vi "Config.vi"() -> ()   [LabVIEW 2020]
uses:
  Global_Variable/A131258.vi
  Global_Variable/Global.vi
  Database/Global1.vi
  <vilib>/Utility/config.llb/NI_LVConfig.lvlib
panel:
  in  "工位选择":cluster{"左工位":bool, "右工位":bool}
  in  "系数":bool
  in  "产品型号":string(combo)
  in  "删除":bool
  in  "确定":bool
  in  "添加":bool
  in  "退出":bool
  in  "更新":bool
  in  "选项卡控件":enum32{"产品参数", "系统参数"}(tab)
  in  "判定框范围":string[][](table)=[["°"], ["N"], ["°"], ["N"], ["°"], ["N"], ["°"], ["N"]]
  in  "结果判定参数":string[][](table)=[["N"], ["N"], ["N"], ["N"], ["N"], ["N"], ["N"], ["N"], ["N"]]
  in  "工位滤波":cluster{"启用滤波":bool, "滤波系数":dbl}
  in  "系统参数设置":string[][](table)=[[""], [""], [""], [""]]
  # "上下柱管总成压装"
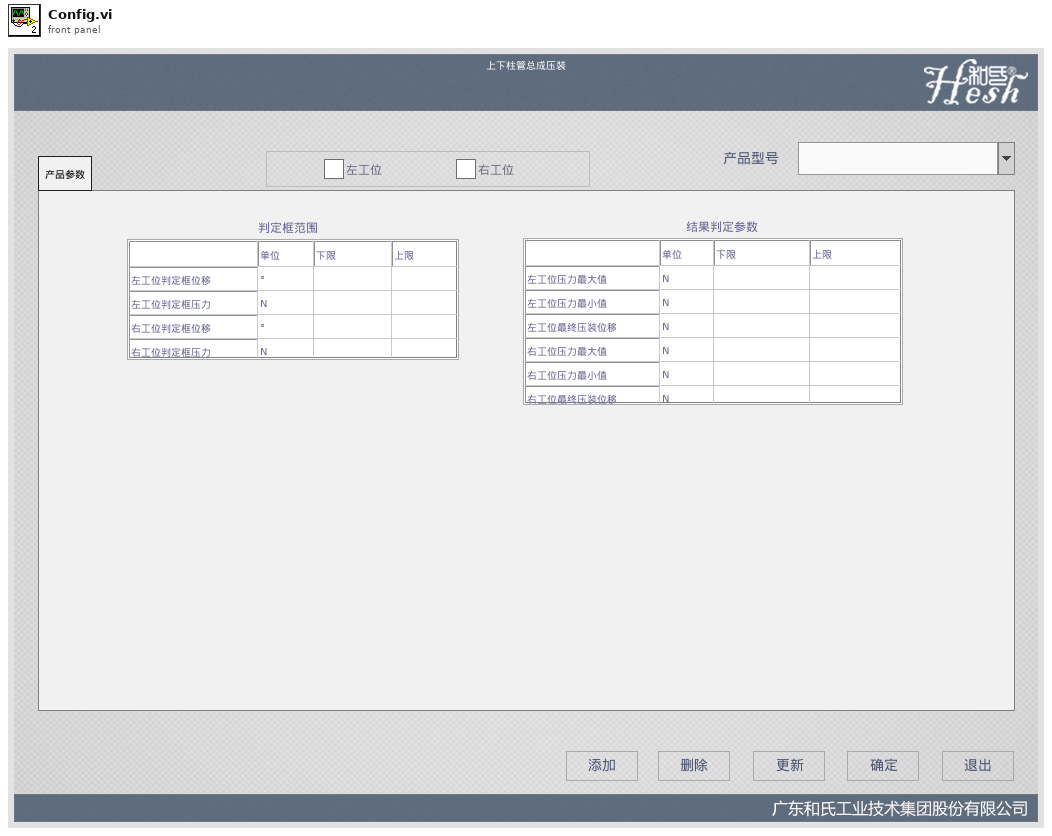
[diagram p1: front panel]
types:
  T1 = typedef "NI_LVConfig.lvlib/Config Data RefNum.ctl" = refnum<k1>
  T2 = cluster{"用户编号":string, "用户名":string, "用户密码(密文)":string, "用户权限":string}
  T3 = cluster{"[0]":cluster{string, dbl, dbl}, "[1]":cluster{string, dbl, dbl}}
  T4 = cluster{"[0]":cluster{string, dbl, dbl}, "[1]":cluster{string, dbl, dbl}, "[2]":cluster{string, dbl, dbl}}
  T5 = cluster{"X ":cluster{"单位":string, "下限":dbl, "上限":dbl}, "Y":cluster{"单位":string, "下限":dbl, "上限":dbl}}
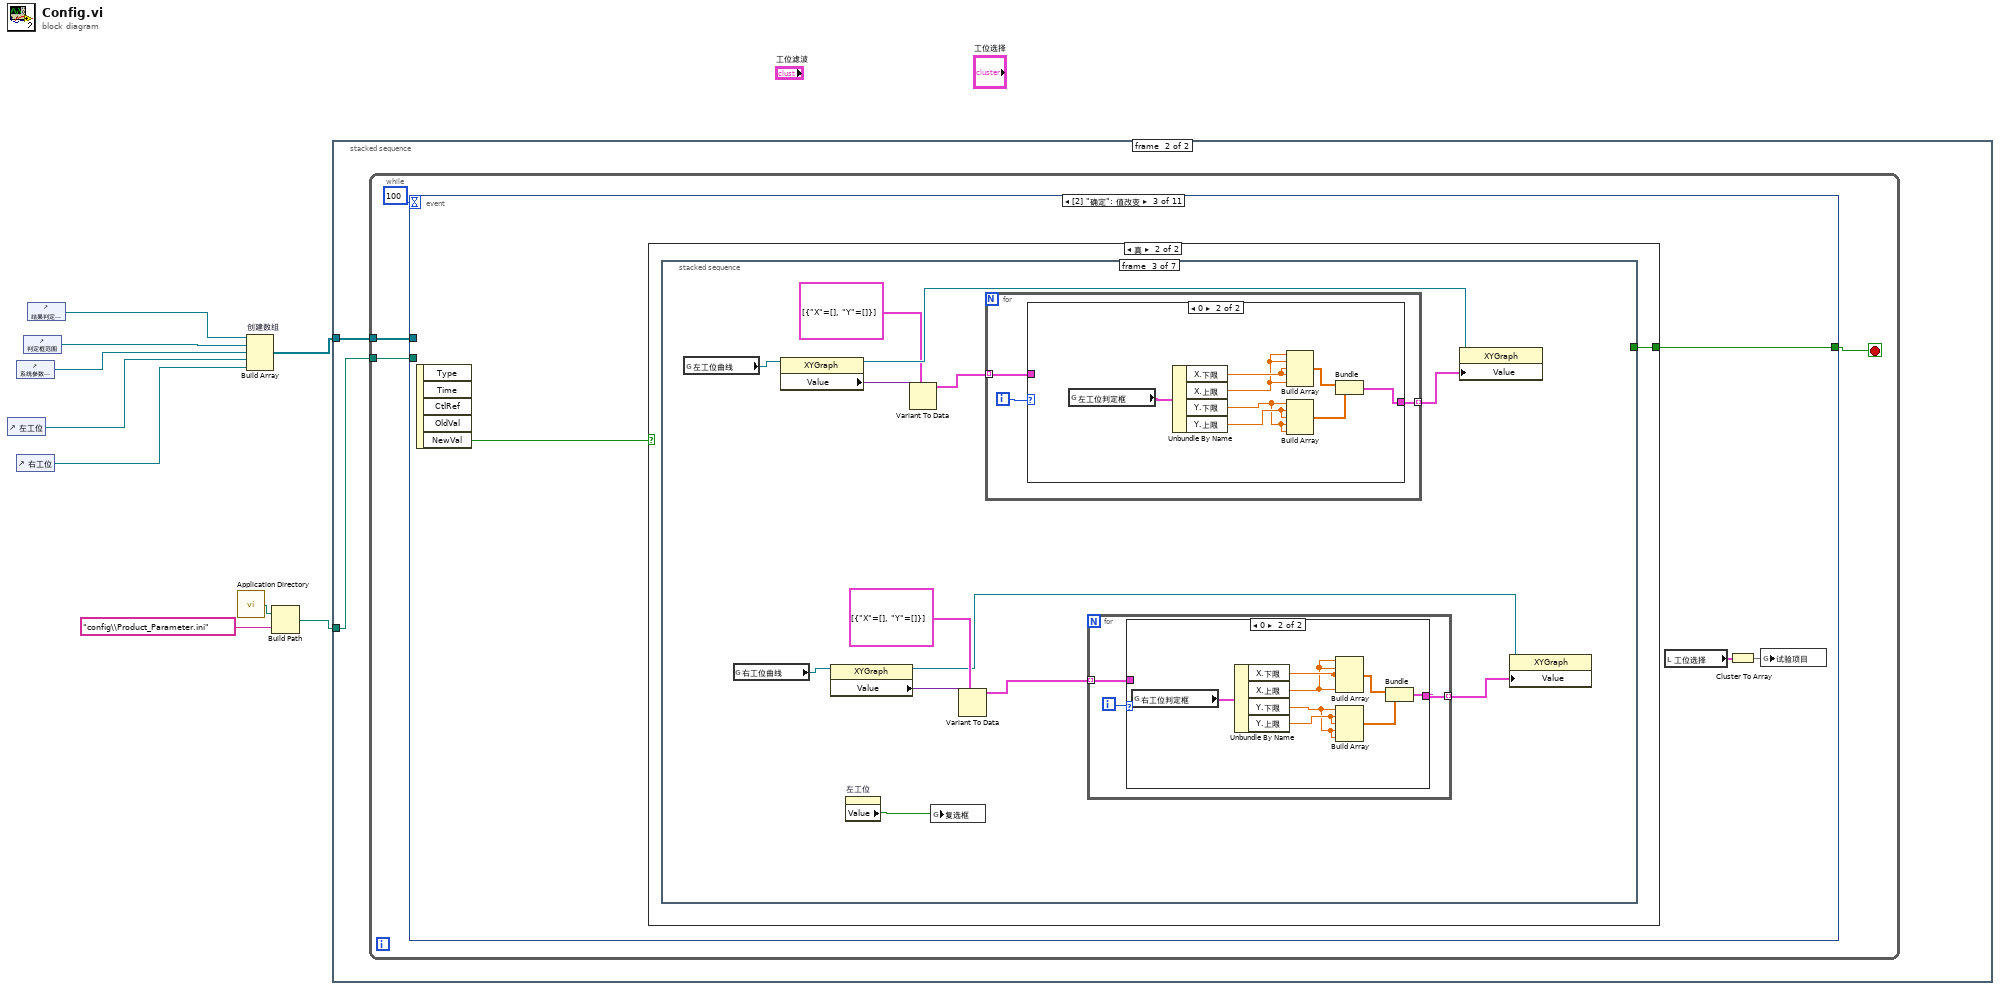
[diagram p0: block diagram]
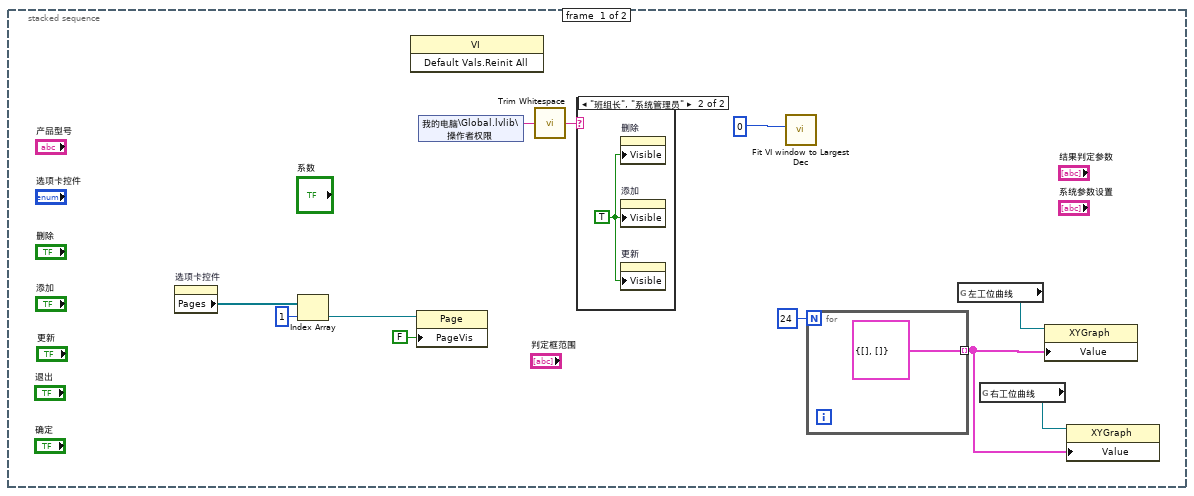
[diagram p2: hidden frame]
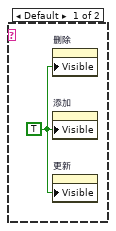
[diagram p3: hidden frame]
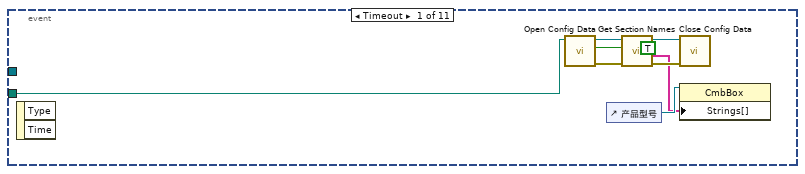
[diagram p4: hidden frame]
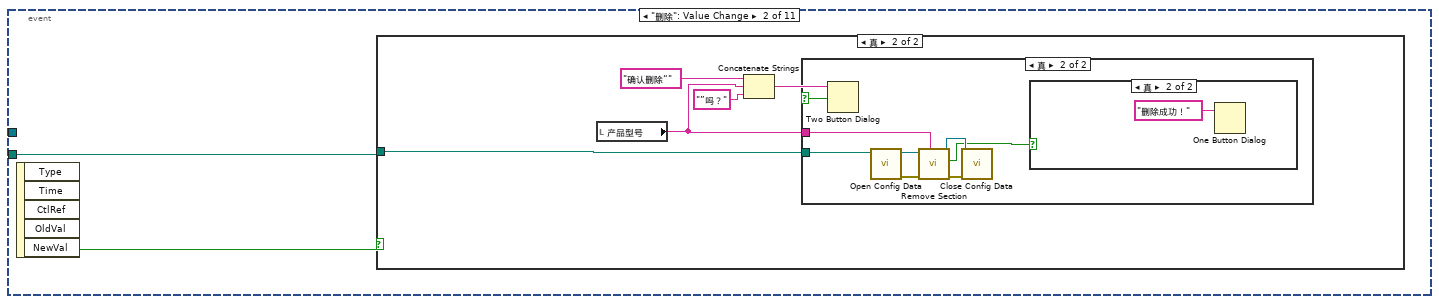
[diagram p5: hidden frame]
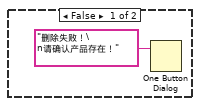
[diagram p8: hidden frame]
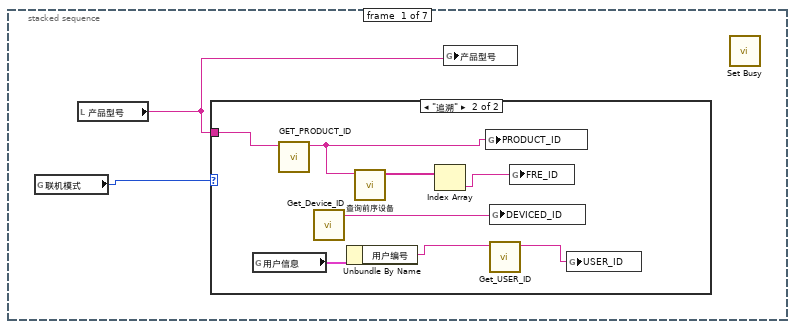
[diagram p10: hidden frame]
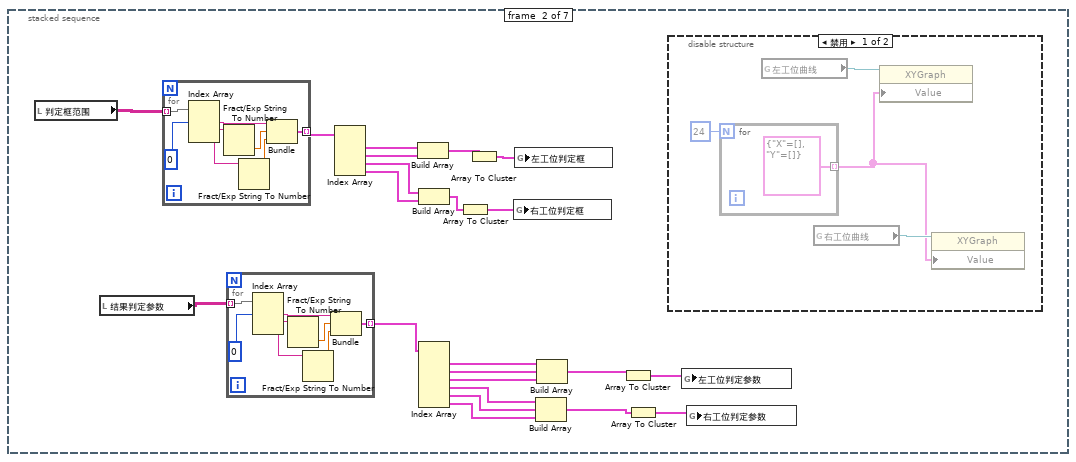
[diagram p12: hidden frame]
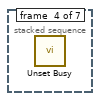
[diagram p16: hidden frame]
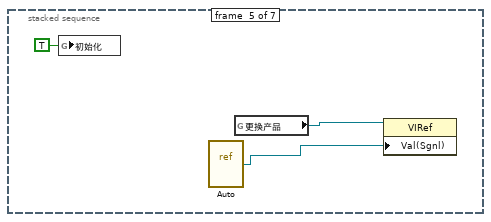
[diagram p17: hidden frame]
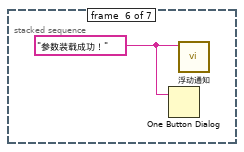
[diagram p18: hidden frame]
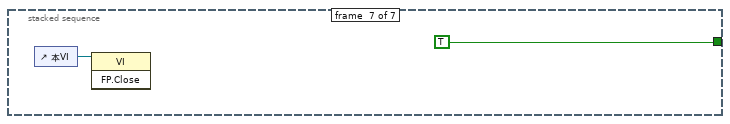
[diagram p19: hidden frame]
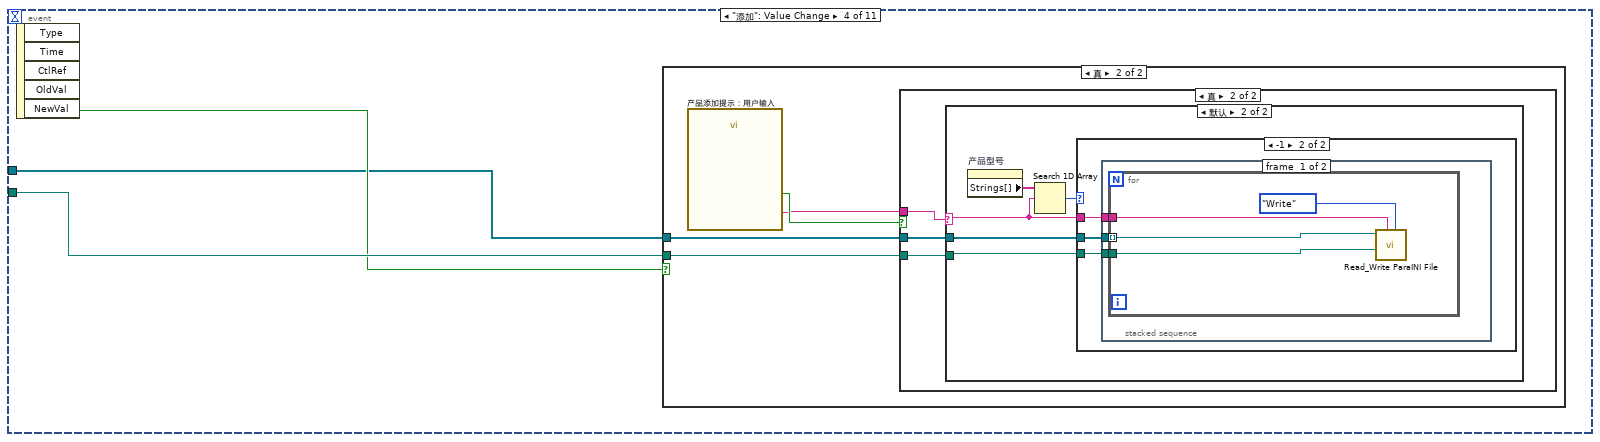
[diagram p20: hidden frame]
diagram:
  n1 = control-ref of="左工位"() -> (w2:refnum<vi>)
  n2 = control-ref of="系统参数设置"() -> (w6:refnum<vi>)
  n3 = control-ref of="右工位"() -> (w1:refnum<vi>)
  n4 = control-ref of="判定框范围"() -> (w3:refnum<vi>)
  n5 = control-ref of="结果判定参数"() -> (w5:refnum<vi>)
  n6 = call <vilib>:"Application Directory.vi"() -> ("Application Directory"=w8:path)
  n7 = Build Array "创建数组"(w5, w3, w6, w2, w1) -> (w9:refnum<vi>[])
  n8 = Build Path(base path=w8, name or relative path="config\\Product_Parameter.ini" ("名称或相对路径")) -> (appended path=w7:path)
  n9 = stacked-sequence {
    tunnel: w9 -> [_ w24]
    tunnel: w7 -> [_ w25]
    frame #0 {
      n10 = property on="选项卡控件" class="TabCtl (严格)"() -> ("Pages"=w16:refnum<vi>[])  [unwired: 2 in, 2 out]
      n11 = Index Array(array=w16, index=1 ("索引")) -> (element=w17:refnum<vi>)
      n12 = invoke class="VI" method="Default Vals.Reinit All"() -> ()  [unwired: 3 in, 3 out]
      n13 = property class="Page"(reference=w17, "PageVis"=FALSE ("选项卡可见")) -> ()  [unwired: 1 in, 2 out]
      n14 = shared-variable "我的电脑\\Global.lvlib\\操作者权限"() -> (w20:string)  [unwired: 1 in, 1 out]
      n15 = call <vilib>:"Trim Whitespace.vi"("string"=w20) -> ("trimmed string"=w19:string)  [unwired: 1 in]
      n16 = case shown="\"班组长\", \"系统管理员\"" w19 {
        frame Default {
          w22 = TRUE ("可见")
          n17 = property on="删除" class="Bool (严格)"("Visible"=w22) -> ()  [unwired: 2 in, 2 out]
          n18 = property on="添加" class="Bool (严格)"("Visible"=w22) -> ()  [unwired: 2 in, 2 out]
          n19 = property on="更新" class="Bool (严格)"("Visible"=w22) -> ()  [unwired: 2 in, 2 out]
        }
        frame "班组长", "系统管理员" {
          w23 = TRUE ("可见")
          n20 = property on="删除" class="Bool (严格)"("Visible"=w23) -> ()  [unwired: 2 in, 2 out]
          n21 = property on="添加" class="Bool (严格)"("Visible"=w23) -> ()  [unwired: 2 in, 2 out]
          n22 = property on="更新" class="Bool (严格)"("Visible"=w23) -> ()  [unwired: 2 in, 2 out]
        }
      }
      n23 = call "Fit VI window to Largest Dec.vi"("border spacing (2 px)"=0) -> ()  [unwired: 5 in, 2 out]
      n24 = for {
        N: 24 -> [_]
        tunnel: [cluster{dbl[], dbl[]} {[], []}] -> w10 mode=indexing
      }
      n25 = global read "A131258.vi" "左工位曲线"() -> (w12:refnum<vi>)
      n26 = global read "A131258.vi" "右工位曲线"() -> (w11:refnum<vi>)
      n27 = property class="XYGraph"(reference=w12, "Value"=w10) -> ()  [unwired: 1 in, 2 out]
      n28 = property class="XYGraph"(reference=w11, "Value"=w10) -> ()  [unwired: 1 in, 2 out]
    }
    frame #1 {
      n29 = while {
        tunnel: w25 -> [w29]
        tunnel: w24 -> [w26]
        stop <- w28 stop-if-true
        n30 = event shown="[2] \"确定\": 值改变" {
          selector: _ -> [_ _ _ _ _ _ _ _ _ _ _]
          dyn-events: _ -> [_ _ _ _ _ _ _ _ _ _ _]
          timeout: 100 -> [_ _ _ _ _ _ _ _ _ _ _]
          tunnel: w29 -> [w30 w39 _ w158 w186 _ w209 _ _ _ _]
          tunnel: [_ _ w57 _ _ TRUE _ _ _ _ TRUE] -> w28
          tunnel: w26 -> [_ _ _ w156 w184 _ w207 _ _ _ _]
          event Timeout {
            n31 = event-data() -> ()  [unwired: 1 in, 2 out]
            n32 = call <vilib>:"Open Config Data.vi"("create file if necessary (T)"=TRUE, "configuration file path"=w30) -> ("error out"=w34:errorcluster, "refnum"=w33:T1)  [unwired: 7 in, 1 out]
            n33 = control-ref of="产品型号"() -> (w32:refnum<vi>)
            n34 = call <vilib>:"Get Section Names.vi"("error in (no error)"=w34, "refnum"=w33) -> ("error out"=w36:errorcluster, "section names"=w31:string[], "refnum out"=w35:T1)  [unwired: 7 in]
            n35 = call <vilib>:"Close Config Data.vi"("error in (no error)"=w36, "refnum"=w35) -> ()  [unwired: 8 in, 2 out]
            n36 = property on="属性节点" class="CmbBox"(reference=w32, "Strings[]"=w31) -> ()  [unwired: 1 in, 2 out]
          }
          event "删除": Value Change {
            n37 = event-data() -> ("NewVal"=w38:bool)  [unwired: 1 in, 4 out]
            n38 = case shown="真" w38 {
              tunnel: w39 -> [_ w41]
              frame False {
              }
              frame True {
                n39 = local read "产品型号"() -> (w40:string)
                n40 = Concatenate Strings("确认删除“", w40, "”吗？") -> (w43:string)
                n41 = Two Button Dialog(message=w43) -> (T button?=w42:bool)  [unwired: 2 in]
                n42 = case shown="真" w42 {
                  tunnel: w41 -> [_ w47]
                  tunnel: w40 -> [_ w46]
                  frame False {
                  }
                  frame True {
                    n43 = call <vilib>:"Open Config Data.vi"("configuration file path"=w47) -> ("error out"=w49:errorcluster, "refnum"=w52:T1)  [unwired: 8 in, 1 out]
                    n44 = call <vilib>:"Remove Section.vi"("section"=w46, "error in (no error)"=w49, "refnum"=w52) -> ("error out"=w51:errorcluster, "section exists?"=w48:bool, "refnum out"=w50:T1)  [unwired: 6 in]
                    n45 = call <vilib>:"Close Config Data.vi"("error in (no error)"=w51, "refnum"=w50) -> ()  [unwired: 8 in, 2 out]
                    n46 = case shown="真" w48 {
                      frame False {
                        n47 = One Button Dialog(message="删除失败！\n请确认产品存在！" ("消息")) -> ()  [unwired: 1 in, 1 out]
                      }
                      frame True {
                        n48 = One Button Dialog(message="删除成功！" ("消息")) -> ()  [unwired: 1 in, 1 out]
                      }
                    }
                  }
                }
              }
            }
          }
          event "确定": Value Change {
            n49 = event-data() -> ("NewVal"=w58:bool)  [unwired: 1 in, 4 out]
            n50 = case shown="真" w58 {
              tunnel: [_ w59] -> w57
              frame False {
              }
              frame True {
                n51 = stacked-sequence {
                  tunnel: [_ _ _ _ _ _ TRUE] -> w59
                  frame #0 {
                    n52 = global read "Global1.vi" "联机模式"() -> (w61:enum16{"单机", "追溯"})
                    n53 = local read "产品型号"() -> (w60:string)
                    n54 = case shown="\"追溯\"" w61 {
                      tunnel: w60 -> [_ w69]
                      frame "单机", Default {
                      }
                      frame "追溯" {
                        n55 = global read "Global1.vi" "用户信息"() -> (w67:T2)
                        n56 = call "GET_PRODUCT_ID.vi"("PRODFUCT_NAME"=w69) -> ("PRODUCT_ID"=w65:string)  [unwired: 10 in]
                        n57 = call "Get_Device_ID.vi"() -> ("Device_ID"=w63:string)  [unwired: 10 in, 1 out]
                        n58 = Unbundle By Name(w67) -> ("用户编号"=w66:string)
                        n59 = call "查询前序设备.vi"("PRODUCT_ID"=w65) -> ("前序工位"=w68:string[])  [unwired: 10 in]
                        n60 = Index Array(array=w68) -> (element=w64:string)  [unwired: 1 in]
                        n61 = global write "Global.vi" "PRODUCT_ID"(w65) -> ()
                        n62 = global write "Global.vi" "DEVICED_ID"(w63) -> ()
                        n63 = call "Get_USER_ID.vi"("USER_EMPLOYEE_ID"=w66) -> ("USER_ID"=w62:string)  [unwired: 9 in, 1 out]
                        n64 = global write "Global.vi" "FRE_ID"(w64) -> ()
                        n65 = global write "Global.vi" "USER_ID"(w62) -> ()
                      }
                    }
                    n66 = global write "Global.vi" "产品型号"(w60) -> ()
                    n67 = call <vilib>:"Set Busy.vi"() -> ()  [unwired: 10 in, 2 out]
                  }
                  frame #1 {
                    n68 = local read "判定框范围"() -> (w91:string[][])
                    n69 = local read "结果判定参数"() -> (w90:string[][])
                    n70 = for {
                      tunnel: w91 -> [w108] mode=indexing
                      tunnel: [w110] -> w87 mode=indexing
                      n71 = Index Array(array=w108, index #1=0) -> (element #1=w109:string, element #2=w107:string, element #3=w106:string)  [unwired: 2 in]
                      n72 = Fract/Exp String To Number(string=w107) -> (number=w112:dbl)  [unwired: 3 in, 1 out]
                      n73 = Fract/Exp String To Number(string=w106) -> (number=w111:dbl)  [unwired: 3 in, 1 out]
                      n74 = Bundle(w109, w112, w111) -> (w110:cluster{string, dbl, dbl})  [unwired: 1 in]
                    }
                    n75 = for {
                      tunnel: w90 -> [w100] mode=indexing
                      tunnel: [w102] -> w82 mode=indexing
                      n76 = Index Array(array=w100, index #1=0) -> (element #1=w101:string, element #2=w99:string, element #3=w98:string)  [unwired: 2 in]
                      n77 = Fract/Exp String To Number(string=w99) -> (number=w104:dbl)  [unwired: 3 in, 1 out]
                      n78 = Fract/Exp String To Number(string=w98) -> (number=w103:dbl)  [unwired: 3 in, 1 out]
                      n79 = Bundle(w101, w104, w103) -> (w102:cluster{string, dbl, dbl})  [unwired: 1 in]
                    }
                    n80 = Index Array(array=w87) -> (element #1=w89:cluster{string, dbl, dbl}, element #2=w88:cluster{string, dbl, dbl}, element #3=w77:cluster{string, dbl, dbl}, element #4=w76:cluster{string, dbl, dbl})  [unwired: 4 in]
                    n81 = Build Array(w89, w88) -> (w85:cluster{string, dbl, dbl}[])
                    n82 = Build Array(w77, w76) -> (w75:cluster{string, dbl, dbl}[])
                    n83 = Index Array(array=w82) -> (element #1=w80:cluster{string, dbl, dbl}, element #2=w79:cluster{string, dbl, dbl}, element #3=w74:cluster{string, dbl, dbl}, element #4=w73:cluster{string, dbl, dbl}, element #5=w72:cluster{string, dbl, dbl}, element #6=w71:cluster{string, dbl, dbl})  [unwired: 6 in]
                    n84 = Array To Cluster(array=w75) -> (cluster=w86:T3)
                    n85 = Array To Cluster(array=w85) -> (cluster=w84:T3)
                    n86 = global write "Global.vi" "右工位判定框"(w86) -> ()
                    n87 = global write "Global.vi" "左工位判定框"(w84) -> ()
                    n88 = Build Array(w73, w72, w71) -> (w78:cluster{string, dbl, dbl}[])
                    n89 = Build Array(w80, w79, w74) -> (w81:cluster{string, dbl, dbl}[])
                    n90 = Array To Cluster(array=w81) -> (cluster=w83:T4)
                    n91 = Array To Cluster(array=w78) -> (cluster=w70:T4)
                    n92 = disable-structure shown="禁用" {
                      frame Disabled {
                        n93 = for {
                          N: 24 -> [_]
                          tunnel: [cluster{"X":dbl[], "Y":dbl[]} {"X"=[], "Y"=[]}] -> w92 mode=indexing
                        }
                        n94 = global read "A131258.vi" "左工位曲线"() -> (w95:refnum<vi>)
                        n95 = global read "A131258.vi" "右工位曲线"() -> (w93:refnum<vi>)
                        n96 = property class="XYGraph"(reference=w95, "Value"=w92) -> ()  [unwired: 1 in, 2 out]
                        n97 = property class="XYGraph"(reference=w93, "Value"=w92) -> ()  [unwired: 1 in, 2 out]
                      }
                      frame Enabled {
                      }
                    }
                    n98 = global write "Global.vi" "左工位判定参数"(w83) -> ()
                    n99 = global write "Global.vi" "右工位判定参数"(w70) -> ()
                  }
                  frame #2 {
                    n100 = global read "A131258.vi" "左工位曲线"() -> (w120:refnum<vi>)
                    n101 = global read "A131258.vi" "右工位曲线"() -> (w119:refnum<vi>)
                    n102 = property class="XYGraph"(reference=w120) -> (reference out=w125:refnum<vi>, "Value"=w123:variant)  [unwired: 1 in, 1 out]
                    n103 = property class="XYGraph"(reference=w119) -> (reference out=w114:refnum<vi>, "Value"=w116:variant)  [unwired: 1 in, 1 out]
                    n104 = property on="左工位" class="Bool (严格)"() -> ("Value"=w113:bool)  [unwired: 2 in, 2 out]
                    n105 = Variant To Data(type=cluster{"X":dbl[], "Y":dbl[]}[] [{"X"=[], "Y"=[]}], Variant=w123) -> (data=w122:cluster{"X":dbl[], "Y":dbl[]}[])  [unwired: 1 in, 1 out]
                    n106 = global write "Global.vi" "复选框"(w113) -> ()
                    n107 = Variant To Data(type=cluster{"X":dbl[], "Y":dbl[]}[] [{"X"=[], "Y"=[]}], Variant=w116) -> (data=w117:cluster{"X":dbl[], "Y":dbl[]}[])  [unwired: 1 in, 1 out]
                    n108 = for {
                      tunnel: [w139] -> w124 mode=indexing
                      tunnel: w122 -> [w138] mode=indexing
                      i -> [w140]
                      n109 = case shown="0" w140 {
                        tunnel: [w141 w143] -> w139
                        tunnel: w138 -> [w141 _]
                        frame Default {
                        }
                        frame 0 {
                          n110 = global read "Global.vi" "左工位判定框"() -> (w149:T5)
                          n111 = Unbundle By Name(w149) -> ("X.下限"=w146:dbl, "X.上限"=w142:dbl, "Y.下限"=w147:dbl, "Y.上限"=w148:dbl)
                          n112 = Build Array(w142, w142, w146, w146, w142) -> (w144:dbl[])
                          n113 = Build Array(w147, w148, w148, w147, w147) -> (w145:dbl[])
                          n114 = Bundle(w144, w145) -> (w143:cluster{dbl[], dbl[]})  [unwired: 1 in]
                        }
                      }
                    }
                    n115 = for {
                      tunnel: [w127] -> w115 mode=indexing
                      tunnel: w117 -> [w126] mode=indexing
                      i -> [w128]
                      n116 = case shown="0" w128 {
                        tunnel: [w129 w131] -> w127
                        tunnel: w126 -> [w129 _]
                        frame Default {
                        }
                        frame 0 {
                          n117 = global read "Global.vi" "右工位判定框"() -> (w137:T5)
                          n118 = Unbundle By Name(w137) -> ("X.下限"=w134:dbl, "X.上限"=w130:dbl, "Y.下限"=w135:dbl, "Y.上限"=w136:dbl)
                          n119 = Build Array(w130, w130, w134, w134, w130) -> (w132:dbl[])
                          n120 = Build Array(w135, w136, w136, w135, w135) -> (w133:dbl[])
                          n121 = Bundle(w132, w133) -> (w131:cluster{dbl[], dbl[]})  [unwired: 1 in]
                        }
                      }
                    }
                    n122 = property class="XYGraph"(reference=w125, "Value"=w124) -> ()  [unwired: 1 in, 2 out]
                    n123 = property class="XYGraph"(reference=w114, "Value"=w115) -> ()  [unwired: 1 in, 2 out]
                  }
                  frame #3 {
                    n124 = call <vilib>:"Unset Busy.vi"() -> ()  [unwired: 11 in, 1 out]
                  }
                  frame #4 {
                    n125 = global write "Global.vi" "初始化"(TRUE ("初始化")) -> ()
                    n126 = vi-ref "Auto.vi"() -> (w150:refnum<vi>)
                    n127 = global read "Global.vi" "更换产品"() -> (w152:refnum<vi>)
                    n128 = property class="VIRef"(reference=w152, "Val(Sgnl)"=w150) -> ()  [unwired: 1 in, 2 out]
                  }
                  frame #5 {
                    w153 = "参数装载成功！" ("消息")
                    n129 = One Button Dialog(message=w153) -> ()  [unwired: 1 in, 1 out]
                    n130 = call "浮动通知.vi"("通知内容"=w153) -> ()  [unwired: 11 in]
                  }
                  frame #6 {
                    n131 = control-ref of="本VI"() -> (w154:refnum<vi>)
                    n132 = invoke class="VI" method="FP.Close"(reference=w154) -> ()  [unwired: 2 in, 3 out]
                  }
                }
              }
            }
            n133 = local read "工位选择"() -> (w56:cluster{"左工位":bool, "右工位":bool})
            n134 = Cluster To Array(cluster=w56) -> (array=w55:bool[])
            n135 = global write "Global.vi" "试验项目"(w55) -> ()
          }
          event "添加": Value Change {
            n136 = event-data() -> ("NewVal"=w157:bool)  [unwired: 1 in, 4 out]
            n137 = case shown="真" w157 {
              tunnel: w158 -> [_ w162]
              tunnel: w156 -> [_ w159]
              frame False {
              }
              frame True {
                n138 = call "产品添加提示：用户输入"() -> ("产品型号"=w160:string, "确定"=w161:bool)  [unwired: 17 in, 1 out]
                n139 = case shown="真" w161 {
                  tunnel: w162 -> [_ w165]
                  tunnel: w160 -> [_ w164]
                  tunnel: w159 -> [_ w163]
                  frame False {
                  }
                  frame True {
                    n140 = case shown="默认" w164 {
                      selector: w164 -> [_ w169]
                      tunnel: w165 -> [_ w171]
                      tunnel: w163 -> [_ w167]
                      frame "" {
                        n141 = One Button Dialog(message="产品名称不得为空!" ("text")) -> ()  [unwired: 1 in, 1 out]
                      }
                      frame Default {
                        n142 = property on="产品型号" class="CmbBox"() -> ("Strings[]"=w170:string[])  [unwired: 2 in, 2 out]
                        n143 = Search 1D Array(1D array=w170, element=w169) -> (index of element=w168:i32)  [unwired: 1 in]
                        n144 = case shown="-1" w168 {
                          tunnel: w171 -> [_ w175]
                          tunnel: w169 -> [_ w174]
                          tunnel: w167 -> [_ w173]
                          frame Default {
                            n145 = One Button Dialog(message="产品已存在！" ("消息")) -> ()  [unwired: 1 in, 1 out]
                          }
                          frame -1 {
                            n146 = stacked-sequence {
                              tunnel: w175 -> [w178 _]
                              tunnel: w174 -> [w177 _]
                              tunnel: w173 -> [w176 _]
                              frame #0 {
                                n147 = for {
                                tunnel: w178 -> [w182]
                                tunnel: w177 -> [w179]
                                tunnel: w176 -> [w181] mode=indexing
                                n148 = call "Read_Write ParaINI File.vi"("Mode"=enum16{"Read", "Write"}."Write", "Section"=w179, "Filepath"=w182, "Ctl Refnum"=w181) -> ()  [unwired: 7 in, 1 out]
                                }
                              }
                              frame #1 {
                                n149 = One Button Dialog(message="添加成功！" ("消息")) -> ()  [unwired: 1 in, 1 out]
                              }
                            }
                          }
                        }
                      }
                    }
                  }
                }
              }
            }
          }
          event "产品型号": Value Change {
            n150 = event-data() -> ("NewVal"=w185:string)  [unwired: 1 in, 4 out]
            n151 = stacked-sequence {
              tunnel: w186 -> [_ _ w190]
              tunnel: w185 -> [_ w188 _]
              tunnel: w184 -> [_ _ w189]
              frame #0 {
                n152 = control-ref of="本VI"() -> (w187:refnum<vi>)
                n153 = invoke class="VI" method="Default Vals.Reinit All"(reference=w187) -> ()  [unwired: 2 in, 3 out]
              }
              frame #1 {
                n154 = local write "产品型号"(w188) -> ()
              }
              frame #2 {
                n155 = disable-structure shown="启用" {
                  disable-tunnel: w190 -> [w191 w199]
                  disable-tunnel: w189 -> [_ w200]
                  frame Disabled {
                    n156 = for {
                      tunnel: [w195] -> w192 mode=indexing
                      tunnel: w191 -> [w194]
                      n157 = local read "产品型号"() -> (w193:string)
                      n158 = call "Read_Write ParaINI File.vi"("Mode"=enum16{"Read", "Write"}."Read", "Section"=w193, "Filepath"=w194, "Ctl Refnum"=w195) -> ()  [unwired: 7 in, 1 out]
                    }
                  }
                  frame Enabled {
                    n159 = local read "产品型号"() -> (w201:string)
                    n160 = call <vilib>:"Set Busy.vi"() -> ("error out"=w198:errorcluster)  [unwired: 10 in, 1 out]
                    n161 = call "Read_Write INI File.vi"("Mode"=enum16{"Read", "Write"}."Read", "Section"=w201, "error in"=w198, "Filepath"=w199, "Ctl Refnum"=w200) -> ("error out"=w197:errorcluster)  [unwired: 6 in]
                    n162 = call <vilib>:"Unset Busy.vi"("error in (no error)"=w197) -> ()  [unwired: 10 in, 1 out]
                  }
                }
              }
            }
          }
          event "退出": Value Change {
            n163 = event-data() -> ()  [unwired: 1 in, 5 out]
            n164 = control-ref of="本VI"() -> (w205:refnum<vi>)
            n165 = invoke class="VI" method="FP.Close"(reference=w205) -> (reference out=w203:refnum<vi>, error out=w204:errorcluster)  [unwired: 2 in, 1 out]
            n166 = Close Reference(reference=w203, error in (no error)=w204) -> ()  [unwired: 1 out]
          }
          event "更新": Value Change {
            n167 = event-data() -> ("NewVal"=w208:bool)  [unwired: 1 in, 4 out]
            n168 = case shown="真" w208 {
              tunnel: w209 -> [_ w212]
              tunnel: w207 -> [_ w210]
              frame False {
              }
              frame True {
                n169 = for {
                  tunnel: w212 -> [w219]
                  tunnel: [w218] -> w211
                  tunnel: w210 -> [w217] mode=indexing
                  n170 = local read "产品型号"() -> (w221:string)
                  n171 = call "Read_Write ParaINI File.vi"("Mode"=enum16{"Read", "Write"}."Write", "Section"=w221, "Filepath"=w219, "Ctl Refnum"=w217) -> ("error out"=w218:errorcluster)  [unwired: 7 in]
                }
                n172 = case shown="无错误" w211 {
                  frame No Error {
                    n173 = Wait (ms)(milliseconds to wait=u32 500 ("等待时间（毫秒）")) -> ()  [unwired: 1 out]
                    n174 = One Button Dialog(message="更新成功！" ("通知内容")) -> ()  [unwired: 1 in, 1 out]
                  }
                  frame Error {
                    n175 = Wait (ms)(milliseconds to wait=u32 500 ("等待时间（毫秒）")) -> ()  [unwired: 1 out]
                    n176 = call "浮动通知.vi"("通知内容"="更新失败！") -> ()  [unwired: 11 in]
                  }
                }
              }
            }
          }
          event "系数": Mouse Enter {
            n177 = event-data() -> ()  [unwired: 1 in, 4 out]
            n178 = property on="系数" class="Bool"("Colors [4]"=cluster{u32, u32}[] [{16777216, 16777216}] ("颜色[4]")) -> ()  [unwired: 2 in, 2 out]
          }
          event "系数": Value Change {
            n179 = event-data() -> ("NewVal"=w224:bool)  [unwired: 1 in, 5 out]
            n180 = property on="选项卡控件" class="TabCtl (严格)"() -> ("Pages"=w226:refnum<vi>[])  [unwired: 2 in, 2 out]
            n181 = Index Array(array=w226, index=1 ("索引")) -> (element=w225:refnum<vi>)
            n182 = property class="Page"(reference=w225, "PageVis"=w224) -> ()  [unwired: 1 in, 2 out]
          }
          event "工位选择.左工位": Value Change {
            n183 = event-data() -> ("NewVal"=w227:bool)  [unwired: 1 in, 5 out]
            n184 = global write "Global.vi" "复选框"(w227) -> ()
          }
          event Panel Close {
            n185 = event-data() -> ()  [unwired: 1 in, 3 out]
          }
        }
      }
    }
  }
